vi "Init Data Object.vi"(11 "ePAS Cell Data in":refnum<class "ePAS Cell Data.lvclass">) -> (3 "ePAS Cell Data out":refnum<class "ePAS Cell Data.lvclass">)   [LabVIEW 2014, in "ePAS Library.lvlib" / "ePAS Cell Data.lvclass"]
uses:
  ePAS Cell Data.lvclass
  reusable/PAS/Data/Cell/PAS Cell Data.lvclass/PAS Cell Data.ctl
  reusable/Data/Data.lvclass/Data.ctl
  reusable/PAS/Data/Cell/PAS Cell Data.lvclass
  reusable/Data/Data.lvclass
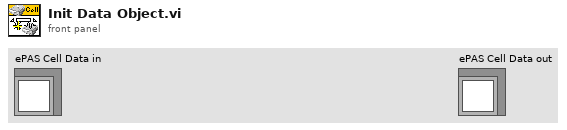
[diagram p1: front panel]
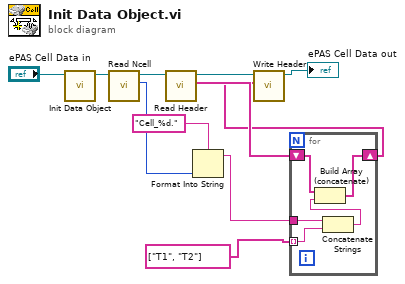
[diagram p0: block diagram]
diagram:
  n1 = call-parent "Init Data Object.vi"("PAS Cell Data in"="ePAS Cell Data in") -> ("PAS Cell Data out"=w10:refnum<class "ePAS Cell Data.lvclass">)  [unwired: 10 in]
  n2 = call "Read Ncell.vi"("PAS Cell Data in"=w10) -> ("Ncell"=w8:u8, "PAS Cell Data out"=w9:refnum<class "ePAS Cell Data.lvclass">)  [unwired: 8 in, 1 out]
  n3 = call "Read Header.vi"("Data in"=w9) -> ("Header"=w6:string[], "Data out"=w2:refnum<class "ePAS Cell Data.lvclass">)  [unwired: 8 in, 1 out]
  n4 = Format Into String(format string="Cell_%d.", w8) -> (resulting string=w4:string)  [unwired: 2 in, 1 out]
  n5 = for {
    shift-right: [w12] -> w3
    shift-left: w6 -> [w16]
    tunnel: string[] ["T1", "T2"] -> [w15] mode=indexing
    tunnel: w4 -> [w14]
    n6 = Concatenate Strings(w14, w15) -> (w13:string)
    n7 = Build Array (concatenate)(w16, w13) -> (w12:string[])
  }
  n8 = call "Write Header.vi"("Header"=w3, "Data in"=w2) -> ("Data out"=→"ePAS Cell Data out":refnum<class "ePAS Cell Data.lvclass">)  [unwired: 8 in, 1 out]
